vi "Disconnect.vi"(8 "error in":errorcluster, 11 "Electronic Load in":refnum<class "Electronic Load.lvclass">) -> (0 "error out":errorcluster, 3 "Electronic Load out":refnum<class "Electronic Load.lvclass">)   [LabVIEW 2019, in "Electronic Load.lvlib" / "Electronic Load.lvclass"]
uses:
  Library/Electronic Load.lvclass
  builds/Instruments/Instruments.lvlibp/Library/Instruments.lvclass
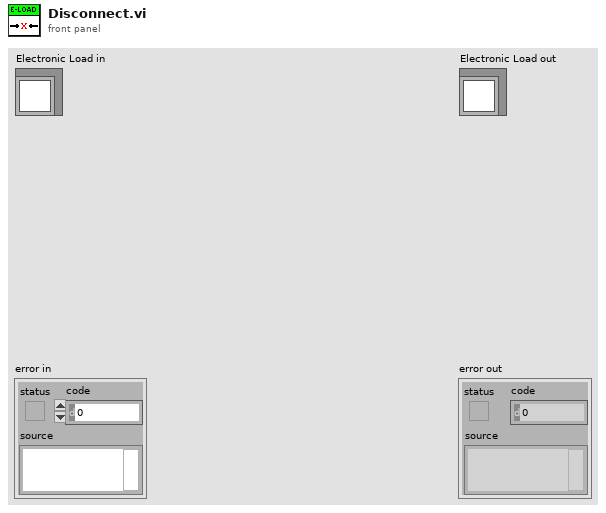
[diagram p1: front panel]
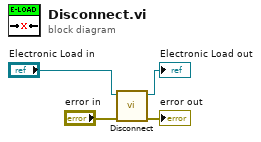
[diagram p0: block diagram]
diagram:
  n1 = call-parent "Disconnect.vi"("error in"="error in", "Instruments in"="Electronic Load in") -> ("error out"=→"error out":errorcluster, "Instruments out"=→"Electronic Load out":refnum<class "Electronic Load.lvclass">)  [unwired: 8 in]
